vi "Read Child Attributes.vi"(11 "TEMPLATE Actor in":refnum<class "TEMPLATE Actor.lvclass">) -> (2 "Child Attributes":T1)   [LabVIEW 2020, in "_Template.lvlib" / "Templates.lvlib" / "TEMPLATE jettl Actor.lvlib" / "TEMPLATE Actor.lvlib" / "TEMPLATE Actor.lvclass"]
uses:
  TEMPLATE Actor.lvclass
  jettl/jettl/Msg/Msg.lvclass
  jettl/jettl/Actor/Actor.lvclass
  jettl/jettl/Transport/Transport.lvclass
  jettl/jettl/Attributes Metadata/Attributes Metadata.lvclass
  TEMPLATE Actor.lvclass/TEMPLATE Actor.ctl
  jettl/jettl/Child Attributes.ctl
  jettl/jettl/jettl.lvlib
  jettl/jettl/Msgs.ctl
  jettl/jettl/Attributes.ctl
panel:
  # "This front panel should not be manipulated."
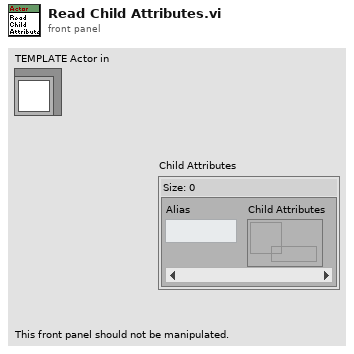
[diagram p1: front panel]
types:
  T1 = typedef "jettl.lvlib/Child Attributes.ctl" = map{string, refnum<data-value>}
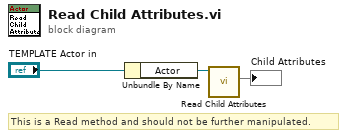
[diagram p0: block diagram]
diagram:
  # "This is a Read method and should not be further manipulated."
  n1 = Unbundle By Name("TEMPLATE Actor in") -> ("Actor"=w2:refnum<class "Actor.lvclass">)
  n2 = call-dynamic "Read Child Attributes.vi"("Actor in"=w2) -> ("Child Attributes"=→"Child Attributes":T1)  [unwired: 10 in]
